vi "Get Device ID.vi"(8 "Error In":errorcluster, 11 "LINX Device Config":T1) -> (0 "Error Out":errorcluster, 2 "Device Name":string, 3 "LINX Device Config":T1)   [LabVIEW 2013, in "LVH-LINX.lvlib" / "Device.lvlib"]
uses:
  <vilib>/LabVIEW Hacker/LINX/Private/Device/Device.lvlib
  <vilib>/LabVIEW Hacker/LINX/Private/Device/Type Defs/LINX Device Config.ctl
  <vilib>/LabVIEW Hacker/LINX/Private/Type Defs/Interface.ctl
  <vilib>/LabVIEW Hacker/LINX/Private/Device/Type Defs/TCP Config.ctl
  <vilib>/LabVIEW Hacker/LINX/Private/Type Defs/Device Family.ctl
  <vilib>/LabVIEW Hacker/LINX/Private/Type Defs/Error Type.ctl
  <vilib>/LabVIEW Hacker/LINX/LVH-LINX.lvlib
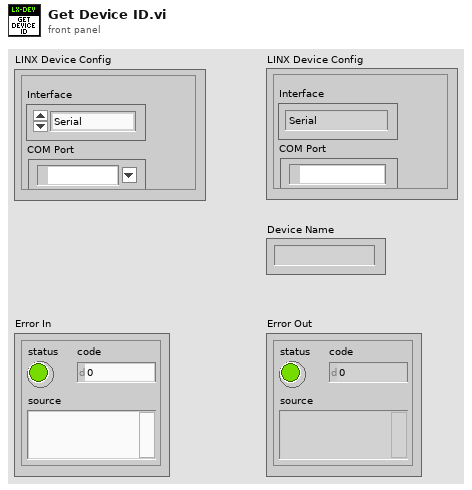
[diagram p1: front panel]
types:
  T1 = typedef "LVH-LINX.lvlib/Device.lvlib/LINX Device Config.ctl" = cluster{"Interface":T2, "COM Port":refnum<visa-resource-name>, "TCP Configuration":T3, "Device Family":T4, "Device ID":u8, "Device Name":string, "TCP Ref":refnum<k5>}
  T2 = typedef "LVH-LINX.lvlib/Interface.ctl" = enum16{"Serial", "TCP"}
  T3 = typedef "LVH-LINX.lvlib/Device.lvlib/TCP Config.ctl" = cluster{"IP Address":string, "Port":u16}
  T4 = typedef "LVH-LINX.lvlib/Device Family.ctl" = enum8{"National Instruments", "Digilent", "Arduino"}
  T5 = typedef "LVH-LINX.lvlib/Error Type.ctl" = enum16{"Unknown", "Timeout", "Corrupt Return Packet", "Unable To Connect", "Command Not Supported", "Channel DNE", "Invalid COM Config"}
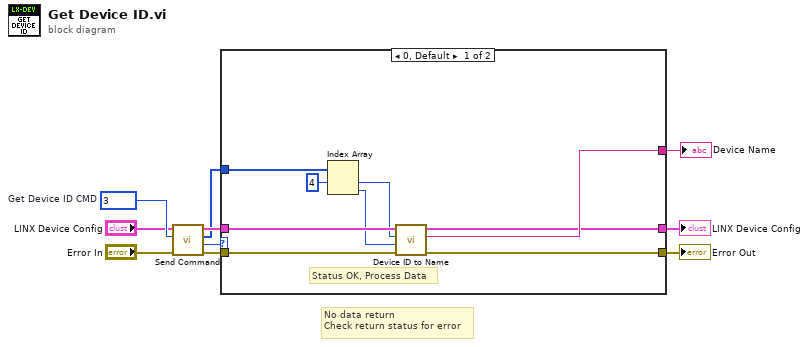
[diagram p0: block diagram]
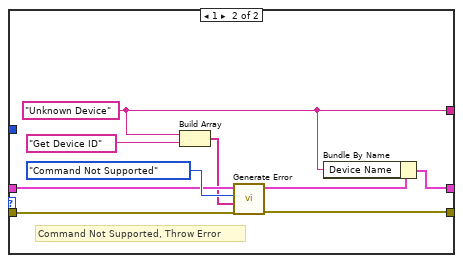
[diagram p2: hidden frame]
diagram:
  w9 = u16 3  # Get Device ID CMD
  # "No data return\nCheck return status for error"
  n1 = call <vilib>:"Send Command.vi"("Error In"="Error In", "CMD"=w9, "LINX Device Config"="LINX Device Config") -> ("Error Out"=w4:errorcluster, "Status"=w1:u8, "Response"=w3:u8[], "LINX Device Config"=w6:T1)  [unwired: 5 in]
  n2 = case shown="0, Default" w1 {
    tunnel: [w11 w21] -> w7
    tunnel: w6 -> [w17 w24]
    tunnel: [w15 w27] -> w5
    tunnel: w4 -> [w16 w28]
    tunnel: w3 -> [w19 _]
    tunnel: [w12 w20] -> w2
    frame 0, Default {
      # "Status OK, Process Data"
      n3 = Index Array(array=w19, index #1=4 ("index")) -> (element #1=w14:u8, element #2=w13:u8)  [unwired: 1 in]
      n4 = call <vilib>:"Device ID to Name.vi"("Error In"=w16, "Device ID"=w13, "Device Family"=w14, "LINX Device Config"=w17) -> ("Error Out"=w15:errorcluster, "Device Name"=w12:string, "LINX Device Config"=w11:T1)  [unwired: 5 in]
    }
    frame 1 {
      w20 = "Unknown Device" ("Device Name")
      # "Command Not Supported, Throw Error"
      n5 = Build Array(w20, "Get Device ID") -> (w23:string[])
      n6 = call <vilib>:"Generate Error.vi"("Error In"=w28, "Arguments"=w23, "Error Type"=Error_Type."Command Not Supported", "LINX Device Config"=w24) -> ("Error Out"=w27:errorcluster, "LINX Device Config"=w22:T1)  [unwired: 6 in]
      n7 = Bundle By Name(cluster=w22, "Device Name"=w20) -> (w21:T1)
    }
  }
  "Error Out" <- w5
  "LINX Device Config" <- w7
  "Device Name" <- w2
